vi "BX.Uninit__LCR.vi"(2 "Container State":T1, 3 "Display State":T2={"Orientation"=0, "ActivePicture"={"image type"=0, "image depth"=0, "image"=[], "mask"=[], "colors"=[], "Rectangle"={"left"=0, "top"=0, "right"=0, "bottom"=0}}, "Pictures"={"Normal"={"image type"=0, "image depth"=0, "image"=[], "mask"=[], "colors"=[], "Rectangle"={"left"=0, "top"=0, "right"=0, "bottom"=0}}, "Hilite"={"image type"=0, "image depth"=0, "image"=[], "mask"=[], "colors"=[], "Rectangle"={"left"=0, "top"=0, "right"=0, "bottom"=0}}}, "Text"={"String"="", "Font"={"Font Name:"="", "Size"=0, "Strikeout?"=FALSE, "Italic?"=FALSE, "Underline?"=FALSE, "Outline?"=FALSE, "Shadow?"=FALSE, "Bold?"=FALSE}, "TextColor"=0}, "RunTimeSettings"={"Highlight"=FALSE, "ShowButton"=TRUE, "Behaviour"=enum."Switch when pressed", "React if disabled"=FALSE, "Nudge Button"=TRUE, "ShowButton on Hover"=FALSE, "Button Type"=enum."System"}, "Messages"=[], "Status"=0, "XControl Label"="", "Boolean Value"=FALSE} {"Status" format="%.0x"}) -> ()   [LabVIEW 2011, in "BooleanXControl__LCR.xctl"]
uses:
  BooleanXControl__LCR.xctl
  BX.State__LCR.ctl
  Controls/BX.Orientation__LCR.ctl
  <vilib>/picture/picture.llb/imagedata.ctl
  Controls/BX.RTSettings__LCR.ctl
  Controls/BX.Behaviour__LCR.ctl
  Controls/BX.ButtonType__LCR.ctl
  Controls/BX.Message__LCR.ctl
  Controls/BX.Commands__LCR.ctl
  <vilib>/_xctls/Container State.ctl
  <vilib>/_xctls/XControlSupport.lvlib
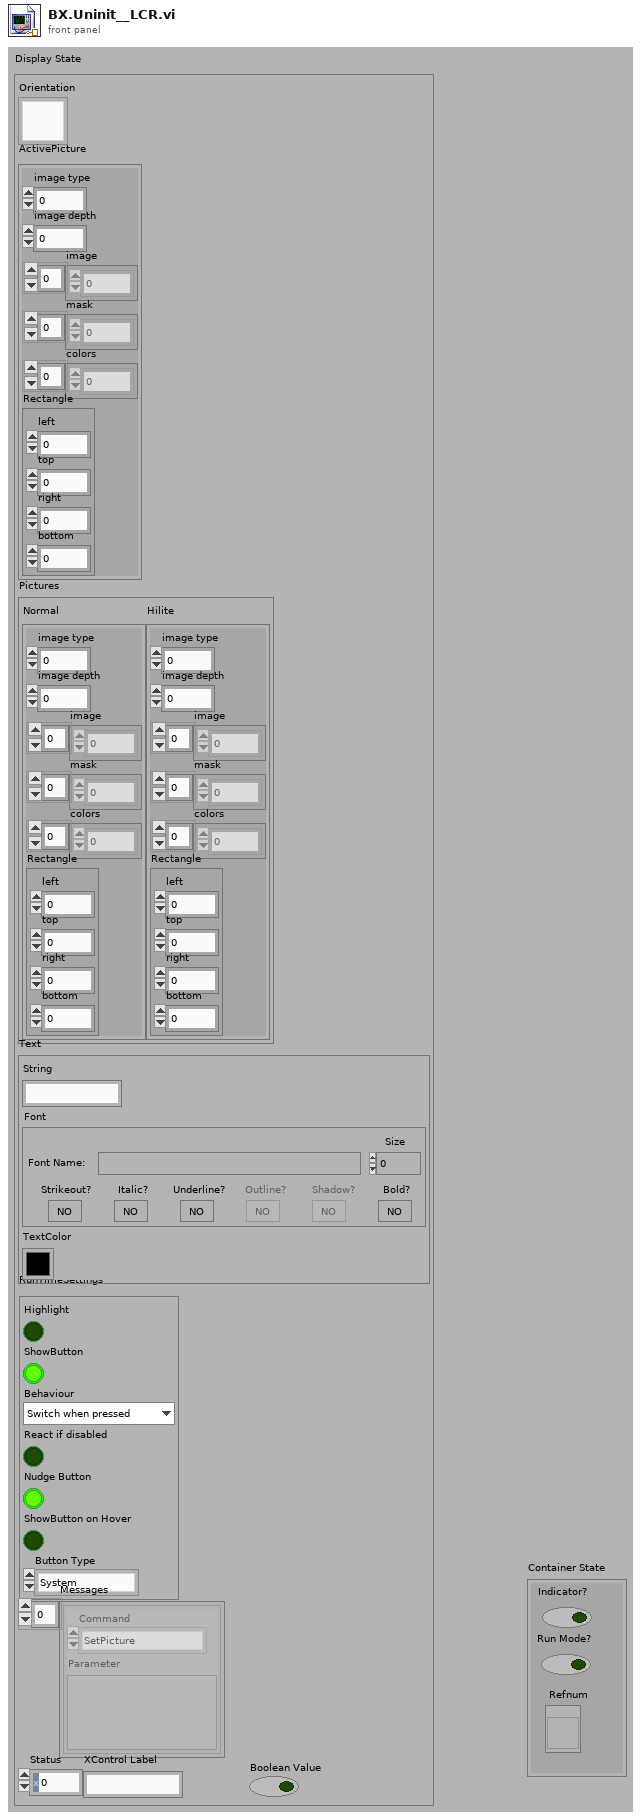
[diagram p1: front panel]
types:
  T1 = typedef "XControlSupport.lvlib/Container State.ctl" = cluster{"Indicator?":bool, "Run Mode?":bool, " Refnum":refnum<vi>}
  T2 = typedef "BooleanXControl__LCR.xctl/BX.State__LCR.ctl" = cluster{"Orientation":T3, "ActivePicture":T4, "Pictures":cluster{"Normal":T4, "Hilite":T4}, "Text":cluster{"String":string, "Font":cluster{"Font Name:":string, "Size":i16, "Strikeout?":bool, "Italic?":bool, "Underline?":bool, "Outline?":bool, "Shadow?":bool, "Bold?":bool}, "TextColor":u32}, "RunTimeSettings":T5, "Messages":T8[], "Status":u16, "XControl Label":string, "Boolean Value":bool}
  T3 = typedef "BooleanXControl__LCR.xctl/BX.Orientation__LCR.ctl" = u8
  T4 = typedef "imagedata.ctl" = cluster{"image type":i32, "image depth":i32, "image":u8[], "mask":u8[], "colors":u32[], "Rectangle":cluster{"left":i16, "top":i16, "right":i16, "bottom":i16}}
  T5 = typedef "BooleanXControl__LCR.xctl/BX.RTSettings__LCR.ctl" = cluster{"Highlight":bool, "ShowButton":bool, "Behaviour":T6, "React if disabled":bool, "Nudge Button":bool, "ShowButton on Hover":bool, "Button Type":T7}
  T6 = typedef "BooleanXControl__LCR.xctl/BX.Behaviour__LCR.ctl" = enum16{"Switch when pressed", "Switch when released", "Switch until released"}
  T7 = typedef "BooleanXControl__LCR.xctl/BX.ButtonType__LCR.ctl" = enum16{"System", "Modern", "Classic", "Decoration"}
  T8 = typedef "BooleanXControl__LCR.xctl/BX.Message__LCR.ctl" = cluster{"Command":T9, "Parameter":variant}
  T9 = typedef "BooleanXControl__LCR.xctl/BX.Commands__LCR.ctl" = enum16{"None", "SetPicture", "SetFont", "SetText", "SetOrientation", "Redraw", "SetTextColor", "SetRTSettings", "MultipleUpdate", "RT.Button", "RT.Hilite", "RT.Behaviour", "RT.Disabled", "ShowGUI", "RT.Nudge", "RT.Hover", "RT.ButtonType"}
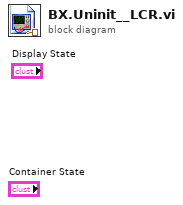
[diagram p0: block diagram]
diagram:
